vi "tsdiag_can_security_access_request_seed.vi"(8 "错误输入（无错误）":errorcluster, 9 "ALevel":i32, 10 "ADiagModuleIndex":i32, 11 "path":path) -> (0 "错误输出":errorcluster, 1 "ARecSeed":u8[](array[numeric]), 2 "Return Type":i32, 3 "path out":path)   [LabVIEW 2014]
doc: "Function Introduction :\n27 seeds to obtain seeds\nCall location :\nAfter connecting the hardware, it is no longer necessary to create a diagnostic module\ninput parameter :\nADiagModulus Index: Handle to UDS module\nALevel: Security Level\nARecSeed: A data pointer used to store seed values\nARecSeedSize: The size of the seed value\nReturn value :\n==0: Execution successful\nOther values: Query error code"
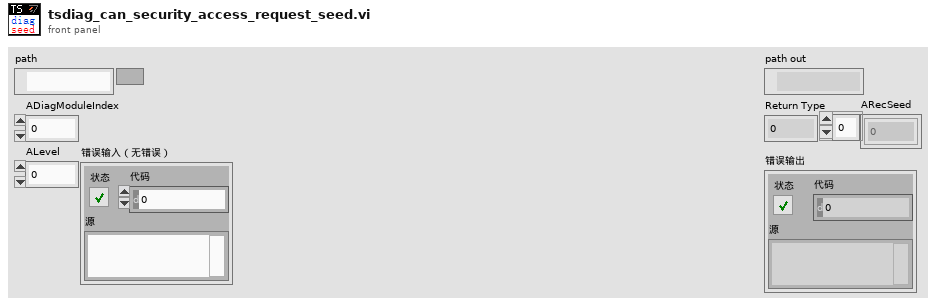
[diagram p1: front panel]
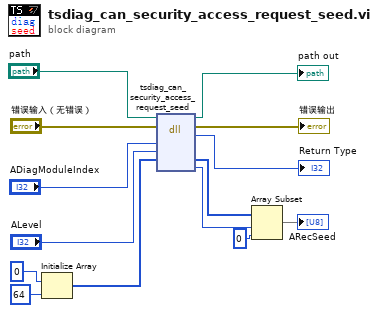
[diagram p0: block diagram]
diagram:
  n1 = Initialize Array(u8 0 ("元素"), 64 ("维数大小")) -> (w8:u8[])
  n2 = dll-call lib="C:/Users/XYY/Desktop/LabView Demo/TSCAN_LB2018_V1.4_20220309/Config/TSMaster.dll" fn="tsdiag_can_security_access_request_seed"(path in="path", error in="错误输入（无错误）", "ADiagModuleIndex"="ADiagModuleIndex", "ALevel"="ALevel", "ARecSeed"=w8) -> (path out=→"path out":path, error out=→"错误输出":errorcluster, "返回类型"=→"Return Type":i32, "ARecSeed"=w3:u8[], "ARecSeedSize"=w2:i32)  [unwired: 4 in]
  n3 = Array Subset(array=w3, index=w2, length=0) -> (→"ARecSeed":u8[])
